vi "Asylum_Driver_RaiseTip.vi"(8 "error in (no error)":errorcluster, 10 "Z Move Setpoint":dbl, 11 "Application In":refnum<k7>) -> (0 "error out":errorcluster, 3 "Application Out":refnum<k7>)   [LabVIEW 2019]
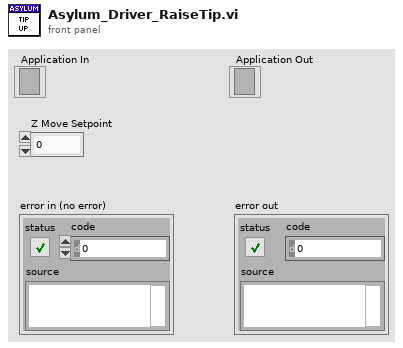
[diagram p1: front panel]
types:
  T1 = cluster{"setpoint":dbl, "pgain":dbl, "igain":dbl, "sgain":dbl}
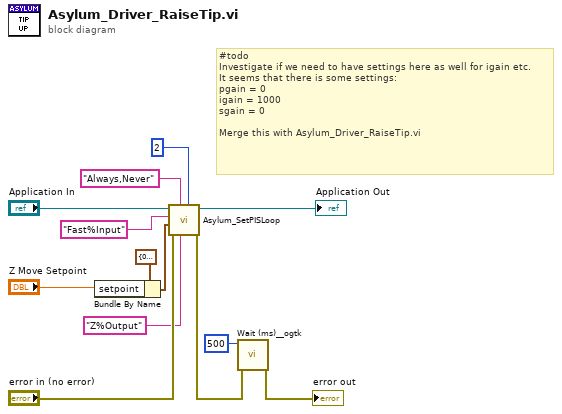
[diagram p0: block diagram]
diagram:
  # "#todo \nInvestigate if we need to have settings here as well for igain etc.\nIt seems that there is some settings:\npgain = 0\nigain = 1000\nsgain = 0\n\nMerge this with Asylum_Driver_RaiseTip.vi"
  n1 = Bundle By Name(cluster=T1 {"setpoint"=0.0, "pgain"=0.0, "igain"=1000.0, "sgain"=0.0} ("PIS Controls"), "setpoint"="Z Move Setpoint") -> (w1:T1)
  n2 = call <userlib>:"Asylum_SetPISLoop.vi"("whichLoop"=2, "outChannelString"="Z%Output", "eventString"="Always,Never", "error in (no error)"="error in (no error)", "PIS Controls"=w1, "inChannelString"="Fast%Input", "Application"="Application In") -> ("error out"=w5:errorcluster, "Application"=→"Application Out":refnum<k7>)  [unwired: 3 in]
  n3 = call <userlib>:"Wait (ms)__ogtk.vi"("error in (no error)"=w5, "milliseconds to wait"=u32 500) -> ("error out"=→"error out":errorcluster)  [unwired: 8 in, 1 out]
